vi "Test Flatten to Path.vi"() -> ()   [LabVIEW 2017]
uses:
  c9b6f366-5878-41eb-ba35-ba660d6be02e.vi
  Variant to JSON Text.vi
  JSONtext.lvlib
panel:
  out "$Paths":string[](array[string])
  out "<JSON>":string
  out "x = y?":bool
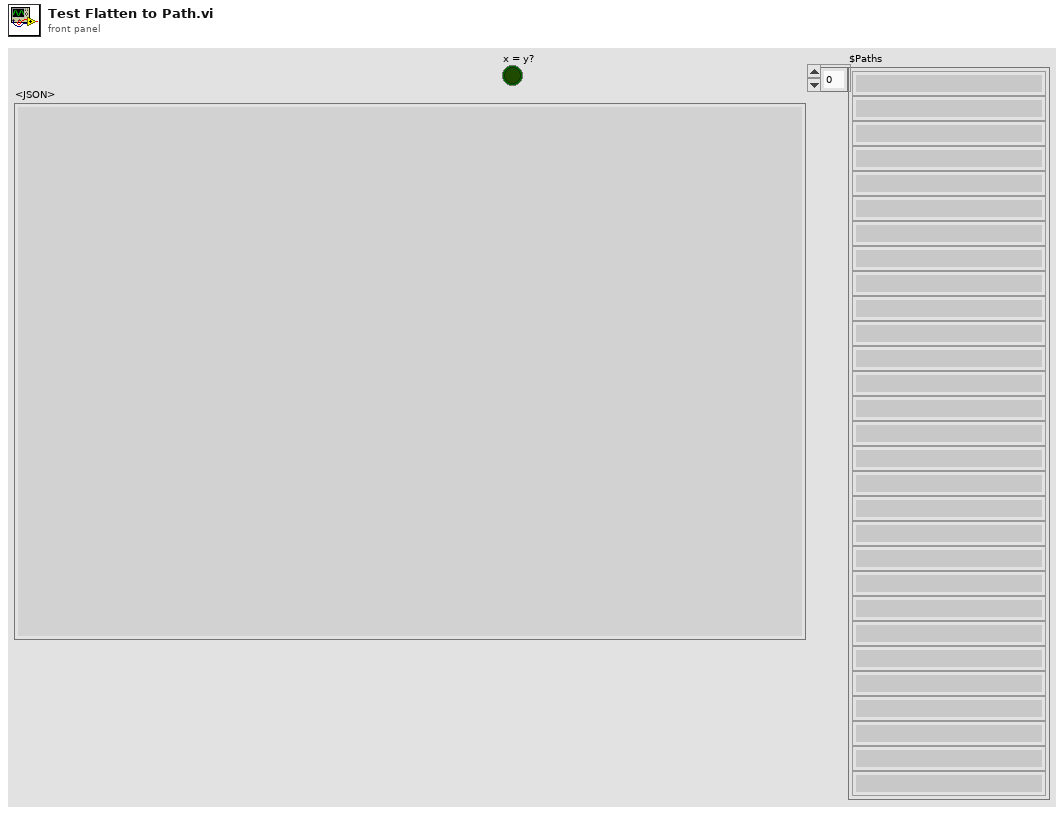
[diagram p1: front panel]
types:
  T1 = cluster{"Number":i32, "String":string, "Timestamp":timestamp, "Reply refnum":refnum<queue>, "VISA resource name":refnum<visa-resource-name>, "True":bool, "Enum":enum16{"Enum 1", "Enum 22", "Enum 333"}, "DBL":dbl, "SubC":cluster{"Number":i32, "String":string, "Timestamp":timestamp, "Reply refnum":refnum<queue>, "VISA resource name":refnum<visa-resource-name>, "True":bool, "Enum":enum16{"Enum 1", "Enum 22", "Enum 333"}, "DBL":dbl, "SubC":cluster{"Number":i32, "String":string, "Timestamp":timestamp, "Reply refnum":refnum<queue>, "VISA resource name":refnum<visa-resource-name>, "True":bool, "Enum":enum16{"Enum 1", "Enum 22", "Enum 333"}, "DBL":dbl}}}
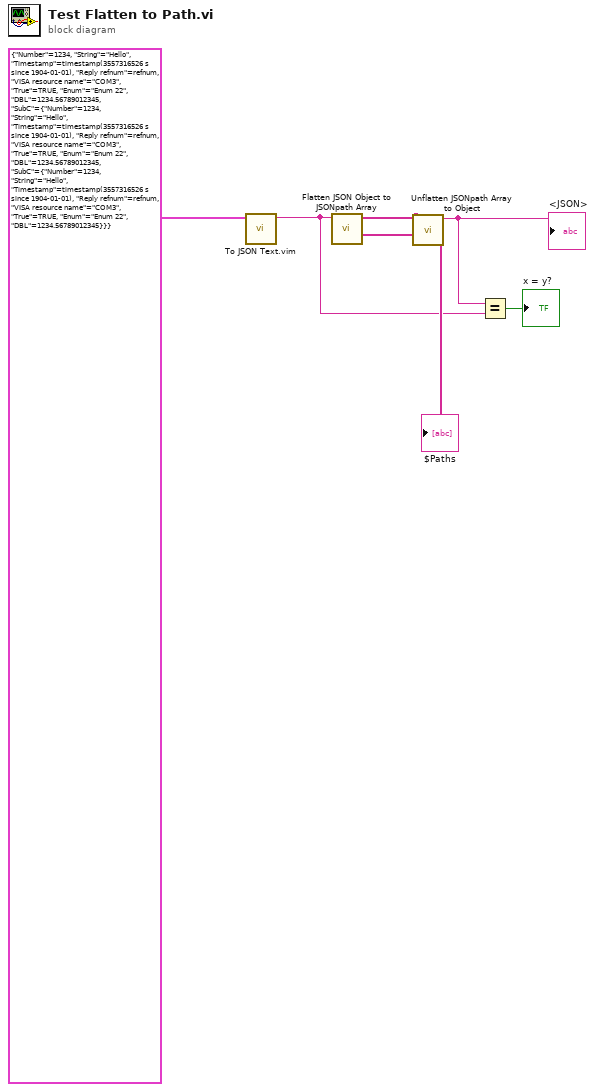
[diagram p0: block diagram]
diagram:
  n1 = call "To JSON Text.vim"("Anything"=T1 {"Number"=1234, "String"="Hello", "Timestamp"=timestamp(3557316526.864 s since 1904-01-01), "Reply refnum"=refnum, "VISA resource name"="COM3", "True"=TRUE, "Enum"=enum."Enum 22", "DBL"=1234.56789012345, "SubC"={"Number"=1234, "String"="Hello", "Timestamp"=timestamp(3557316526.864 s since 1904-01-01), "Reply refnum"=refnum, "VISA resource name"="COM3", "True"=TRUE, "Enum"=enum."Enum 22", "DBL"=1234.56789012345, "SubC"={"Number"=1234, "String"="Hello", "Timestamp"=timestamp(3557316526.864 s since 1904-01-01), "Reply refnum"=refnum, "VISA resource name"="COM3", "True"=TRUE, "Enum"=enum."Enum 22", "DBL"=1234.56789012345}}}) -> ("<JSON>"=w3:string)  [unwired: 9 in, 1 out]
  n2 = call "Flatten JSON Object to JSONpath Array.vi"("<JSON> in"=w3) -> ("<JSON>Items"=w1:string[], "$Paths"=w6:string[])  [unwired: 9 in]
  "$Paths" <- w6
  n3 = call "Unflatten JSONpath Array to Object.vi"("<JSON>Items"=w1, "$Paths"=w6) -> ("<JSON>"=w4:string)  [unwired: 8 in, 1 out]
  "<JSON>" <- w4
  n4 = Equal?(x=w4, y=w3) -> (x = y?=→"x = y?":bool)
